vi "fastReadFrames.vi"() -> ()   [LabVIEW 2019]
uses:
  <vilib>/myRIO/Instrument Drivers/Onboard IO/AI/typedefs/AI Reference.ctl
  <vilib>/myRIO/Common/Instrument Driver Framework/Utilities/typedefs/myRIO Generic Hardware Reference.ctl
  <vilib>/myRIO/Common/Instrument Driver Framework/Utilities/typedefs/Hardware Version Enum.ctl
  <vilib>/myRIO/Common/Instrument Driver Framework/Utilities/typedefs/myRIO v1.0 Reference.ctl
  <vilib>/myRIO/Common/Instrument Driver Framework/Utilities/typedefs/Generic FPGA Reference.ctl
  <vilib>/myRIO/Common/Instrument Driver Framework/myRIO v1.0/AI/typedefs/AI Channels List.ctl
  <vilib>/myRIO/Common/Instrument Driver Framework/myRIO v1.0/AI/typedefs/AI Channels Enum.ctl
  <vilib>/myRIO/Common/Instrument Driver Framework/Utilities/typedefs/Analog Scaling Constants List.ctl
  <vilib>/myRIO/Common/Instrument Driver Framework/Utilities/typedefs/Analog Scaling Constants.ctl
  <vilib>/userdefined/High Color/nirio_resource_hc.ctl
  <vilib>/Platform/TimedLoop/XDataNode/timing_clust.ctl
  <vilib>/Platform/TimedLoop/XDataNode/nitl_modes.ctl
  <vilib>/Platform/TimedLoop/XDataNode/wakeup.ctl
  <vilib>/myRIO/Common/Instrument Driver Framework/myRIO v1.0/AI/vis/myRIO v1.1 Open Throughput AI.vi
  <vilib>/Analysis/baseanly.llb/Mean (DBL).vi
  <vilib>/myRIO/Common/Instrument Driver Framework/Utilities/vis/Validate Channels.vi
  <vilib>/myRIO/Common/Instrument Driver Framework/myRIO v1.0/AI/vis/myRIO v1.0 Reserve AI.vi
  <vilib>/myRIO/Common/Instrument Driver Framework/myRIO v1.0/AI/vis/myRIO v1.0 Close AI.vi
  <vilib>/myRIO/Common/Instrument Driver Framework/myRIO v1.0/AI/vis/myRIO v1.0 Build MUX Configuration AI.vi
  <vilib>/myRIO/Common/Instrument Driver Framework/myRIO v1.0/Resource Manager/vis/myRIO v1.0 Reserve Channel List.vi
  <vilib>/myRIO/Common/Instrument Driver Framework/myRIO v1.0/AI/vis/myRIO v1.0 Unreserve AI.vi
  <vilib>/myRIO/Common/Instrument Driver Framework/myRIO v1.0/Resource Manager/vis/myRIO v1.0 Reserve Channel.vi
  <vilib>/myRIO/Common/Instrument Driver Framework/myRIO v1.0/Resource Manager/vis/myRIO v1.0 Unreserve Channel.vi
  <vilib>/myRIO/Common/Instrument Driver Framework/myRIO v1.0/Resource Manager/vis/myRIO v1.0 Unreserve Channel List.vi
  <vilib>/myRIO/Common/Instrument Driver Framework/myRIO v1.0/Resource Manager/vis/myRIO v1.0 Build Mutex Name.vi
  <vilib>/Utility/VariantDataType/GetNumericInfo.vi
  <vilib>/Utility/error.llb/Error Cluster From Error Code.vi
  <vilib>/myRIO/Common/Instrument Driver Framework/myRIO v1.0/myRIO v1.1 Open Throughput.vi
  <vilib>/myRIO/Common/Instrument Driver Framework/myRIO v1.0/AI/vis/myRIO v1.0 Get Scaling Constants AI.vi
  <vilib>/myRIO/Common/Instrument Driver Framework/Utilities/vis/IO Manager.vi
  <vilib>/myRIO/Common/Instrument Driver Framework/Utilities/vis/Configuration Manager.vi
  <vilib>/myRIO/Common/Instrument Driver Framework/myRIO v1.0/myRIO v1.0 Close.vi
  <vilib>/myRIO/Common/Instrument Driver Framework/myRIO v1.0/AI/vis/myRIO v1.0 Read AI.vi
  <vilib>/myRIO/Instrument Drivers/Onboard IO/AI/vis/myRIO AI Open.xnode
  <vilib>/platform/TimedLoop/XDataNode/XDataNode.xnode
  <vilib>/Platform/TimedLoop/XDataNode/XDNodeRunTimeDep.lvlib
  <vilib>/myRIO/Instrument Drivers/Onboard IO/AI/AI.lvlib
  <vilib>/Analysis/NI_AALBase.lvlib
panel:
  out "dt":dbl[](graph)
  out "puste?":bool[](array[boolean])
  out "size(s)":i32[](array[numeric])
  in  "Frame length ms":i64=50
  out "dt ramki":u32
  out "Waveform Chart":dbl[][](graph)
  in  "stop":bool
  in  "Channel Names":tag[](array[tag])=["B/AI0", "B/AI1", "B/AI2"]
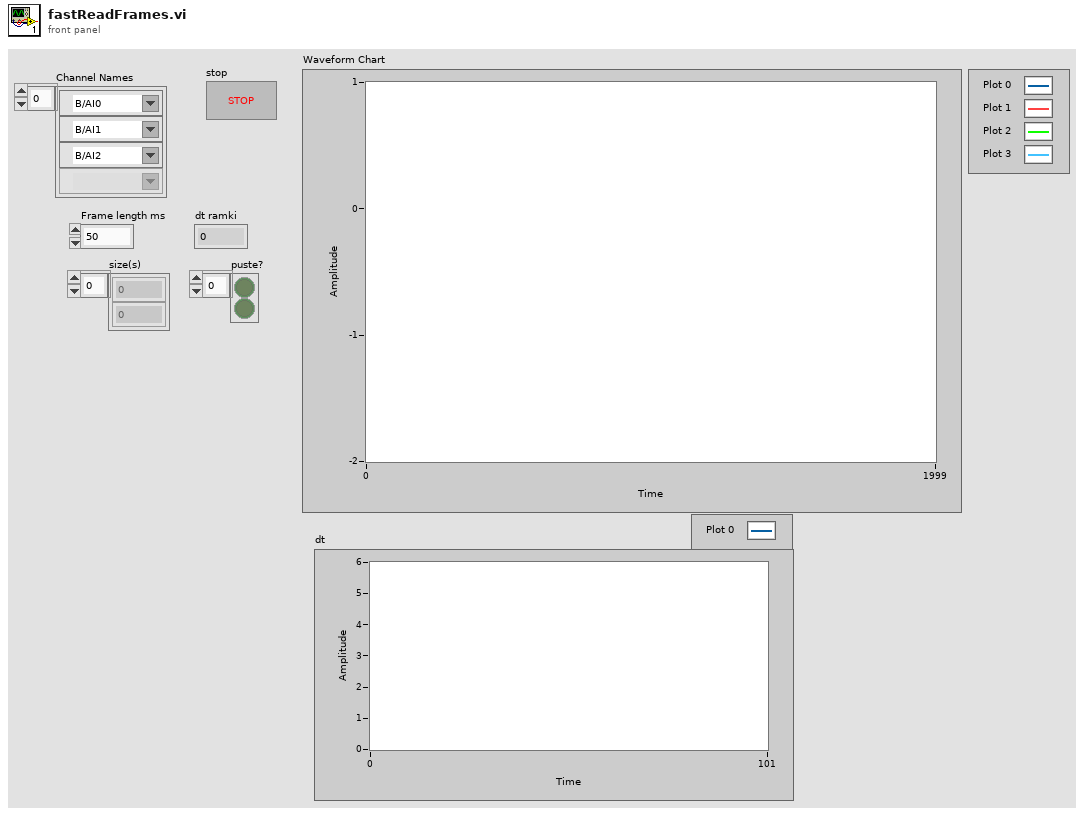
[diagram p1: front panel]
types:
  T1 = typedef "nirio_resource_hc.ctl" = tag
  T2 = typedef "Hardware Version Enum.ctl" = enum16{"Unknown", "myRIO-1900", "myRIO-1950", "roboRIO", "NI ELVIS RIO CM", "ELVIS III"}
  T3 = typedef "AI.lvlib/AI Reference.ctl" = cluster{"myRIO Reference":T4, "AI Channels List":T7, "AI Scaling Constants List":T9}
  T4 = typedef "myRIO Generic Hardware Reference.ctl" = cluster{"myRIO Model":T2, "myRIO Hardware Reference":T5}
  T5 = typedef "myRIO v1.0 Reference.ctl" = cluster{"Generic FPGA Reference":T6, "Allow multiple opens":bool}
  T6 = typedef "Generic FPGA Reference.ctl" = refnum<k20>
  T7 = typedef "AI Channels List.ctl" = T8[]
  T8 = typedef "AI Channels Enum.ctl" = enum16{"Not Connected", "AudioIn/Left", "AudioIn/Right", "C/AI0", "C/AI1", "A/AI0", "A/AI1", "A/AI2", "A/AI3", "A/AI4", "A/AI5", "A/AI6", "A/AI7", "B/AI0", "B/AI1", "B/AI2", "B/AI3", "B/AI4", "B/AI5", "B/AI6", "B/AI7", "AI/AI0", "AI/AI1", "AI/AI2", "AI/AI3", "A/AI0 (DIFF)", "A/AI1 (DIFF)", "A/AI2 (DIFF)", "A/AI3 (DIFF)", "B/AI0 (DIFF)", "B/AI1 (DIFF)", "B/AI2 (DIFF)", "B/AI3 (DIFF)"}
  T9 = typedef "Analog Scaling Constants List.ctl" = T10[]
  T10 = typedef "Analog Scaling Constants.ctl" = cluster{"LSB Weight (Volts)":dbl, "Offset (Volts)":dbl, "Signed?":bool}
  T11 = typedef "XDNodeRunTimeDep.lvlib/timing_clust.ctl" = cluster{"Expected End [f-1]":u64, "Actual End [f-1]":u64, "Finished Late? [f-1]":bool, "Expected End [i-1]":u64, "Actual End [i-1]":u64, "Finished Late? [i-1]":bool, "Expected Start [i]":u64, "Actual Start [i]":u64, "Expected Start [f]":u64, "Actual Start [f]":u64, "Source Name":string, "Structure Name":string, "Period":i64, "Deadline":i64, "Offset":i64, "Start":i64, "Priority":i32, "Timeout":i32, "Mode":T12, "Wakeup Reason":T13, "Error":errorcluster, "Source Type":string, "Secondary Source Type":string, "Global End Time":u64, "Global Start Time":u64, "Frame Duration":u64, "Iteration Duration":u64, "Assigned CPU":i32, "I/O Scan Engine Mode":u32}
  T12 = typedef "XDNodeRunTimeDep.lvlib/nitl_modes.ctl" = enum32{"No Change", "Process missed periods, maintain original phase", "Discard missed periods, maintain original phase", "Process missed periods, ignore original phase", "Discard missed periods, ignore original phase"}
  T13 = typedef "XDNodeRunTimeDep.lvlib/wakeup.ctl" = enum32{"Normal", "Aborted", "Asynchronous wakeup", "Timing source error", "Timed loop error", "Timeout"}
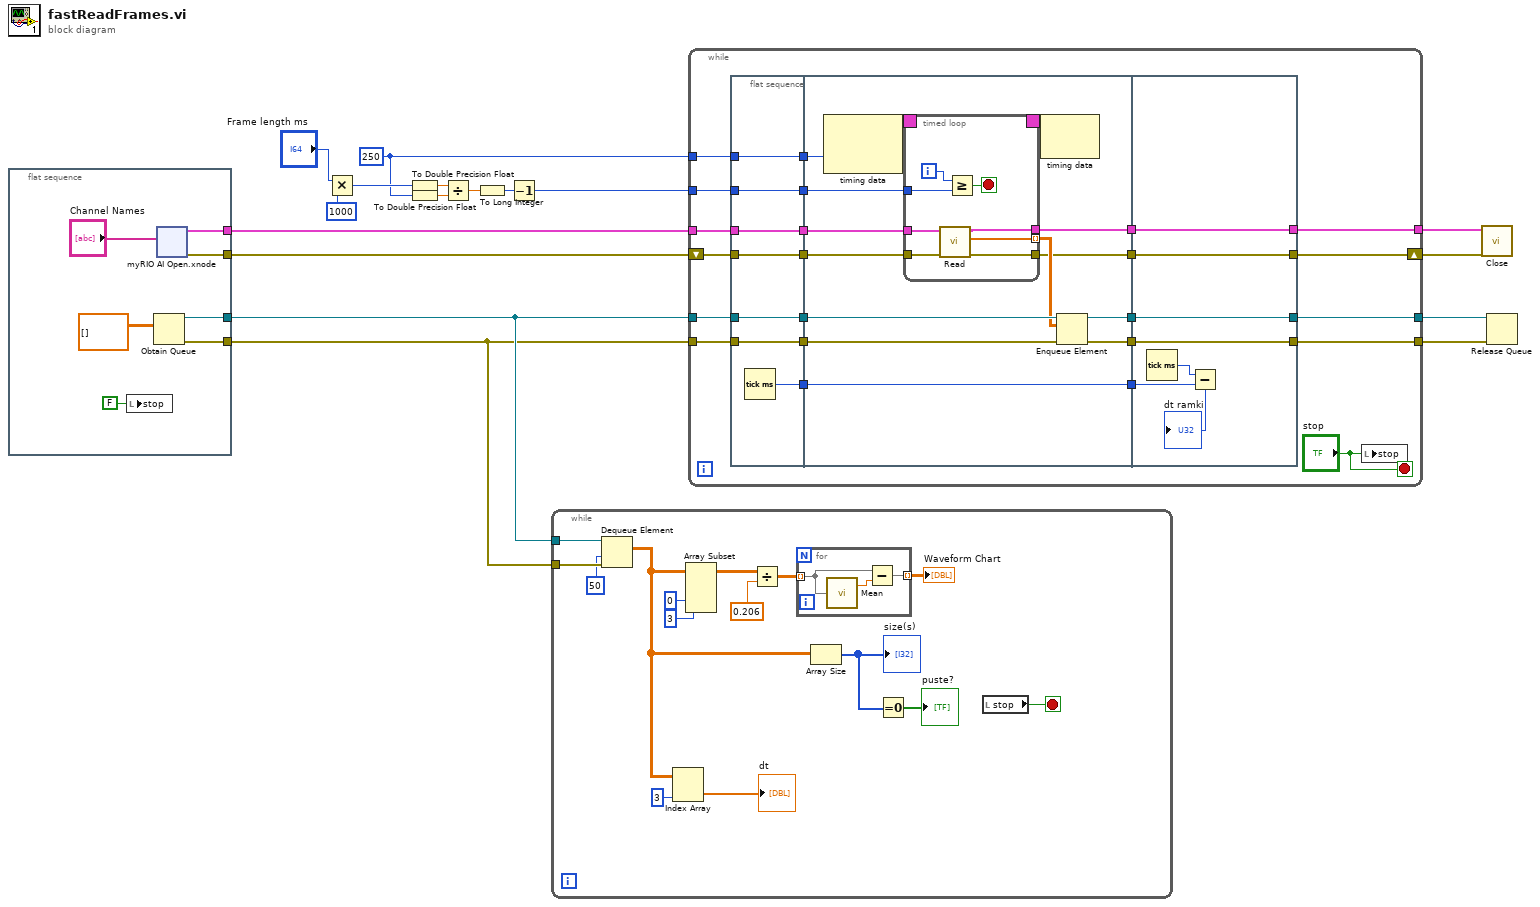
[diagram p0: block diagram]
diagram:
  w3 = i64 250 ("Period")
  n1 = flat-sequence {
    tunnel: [w24] -> w17
    tunnel: [w23] -> w16
    tunnel: [w20] -> w13
    tunnel: [w19] -> w12
    frame #0 {
      n2 = local write "stop"(FALSE ("stop")) -> ()
      n3 = Obtain Queue(element data type=dbl[][] [] ("Values")) -> (queue out=w20:refnum<queue>, error out=w19:errorcluster)  [unwired: 4 in, 1 out]
      n4 = xnode "myRIO AI Open.xnode"("Channel Names"="Channel Names") -> ("error out"=w23:errorcluster, "AI Ref Out"=w24:T3)  [unwired: 2 in]
    }
  }
  n5 = Multiply(x="Frame length ms", y=i64 1000) -> (x*y=w5:i64)
  n6 = To Double Precision Float(number=w5) -> (double precision float=w6:dbl)
  n7 = To Double Precision Float(number=w3) -> (double precision float=w7:dbl)
  n8 = Divide(x=w6, y=w7) -> (x/y=w8:dbl)
  n9 = To Long Integer(number=w8) -> (32bit integer=w9:i32)
  n10 = Decrement(x=w9) -> (x-1=w2:i32)
  n11 = while {
    tunnel: w13 -> [w57]
    tunnel: w12 -> [w56]
    stop <- w54 stop-if-true
    n12 = Dequeue Element(queue=w57, timeout in ms (-1)=50, error in (no error)=w56) -> (element=w45:dbl[][])  [unwired: 3 out]
    n13 = Index Array(array=w45, index (col)=3 ("disabled index (col)")) -> (element=→"dt":dbl[])  [unwired: 1 in]
    n14 = Array Subset(array=w45, index (col)=0 ("index"), length (col)=3 ("length")) -> (w48:dbl[][])  [unwired: 2 in]
    n15 = Divide(x=w48, y=0.206) -> (x/y=w50:dbl[][])
    n16 = for {
      tunnel: w50 -> [w60] mode=indexing
      tunnel: [w59] -> w49 mode=indexing
      n17 = call-poly <vilib>:"Mean.vi"("X"=w60) -> ("mean"=w58:dbl)  [unwired: 1 out]
      n18 = Subtract(x=w60, y=w58) -> (x-y=w59:dbl[])
    }
    "Waveform Chart" <- w49
    n19 = Array Size(array=w45) -> (size(s)=w53:i32[])
    "size(s)" <- w53
    n20 = Equal To 0?(x=w53) -> (x = 0?=→"puste?":bool[])
    n21 = local read "stop"() -> (w54:bool)
  }
  n22 = while {
    tunnel: w17 -> [w83]
    tunnel: w13 -> [w81]
    tunnel: w12 -> [w80]
    tunnel: [w79] -> w15
    tunnel: [w78] -> w14
    tunnel: [w76] -> w11
    shift-right: [w75] -> w10
    shift-left: w16 -> [w82]
    tunnel: w3 -> [w63]
    tunnel: w2 -> [w61]
    stop <- "stop" stop-if-true
    n23 = flat-sequence {
      tunnel: w80 -> [w87]
      tunnel: w81 -> [w88]
      tunnel: w82 -> [w89]
      tunnel: w83 -> [w90]
      tunnel: [w90] -> w74
      tunnel: [w89] -> w73
      tunnel: [w88] -> w72
      tunnel: [w87] -> w71
      tunnel: [w86] -> w70
      tunnel: [w85] -> w64
      tunnel: w63 -> [w85]
      tunnel: [w84] -> w62
      tunnel: w61 -> [w84]
      tunnel: w74 -> [w102]
      tunnel: w73 -> [w101]
      tunnel: w72 -> [w100]
      tunnel: w71 -> [w99]
      tunnel: w70 -> [w93]
      tunnel: [w97] -> w69
      tunnel: [w96] -> w68
      tunnel: [w95] -> w67
      tunnel: [w94] -> w66
      tunnel: [w93] -> w65
      tunnel: w64 -> [w92]
      tunnel: w62 -> [w91]
      tunnel: [w122] -> w75
      tunnel: [w123] -> w76
      tunnel: [w124] -> w78
      tunnel: [w125] -> w79
      tunnel: w69 -> [w125]
      tunnel: w68 -> [w124]
      tunnel: w67 -> [w123]
      tunnel: w66 -> [w122]
      tunnel: w65 -> [w121]
      frame #0 {
        n24 = Tick Count (ms)() -> (millisecond timer value=w86:u32)
      }
      frame #1 {
        n25 = node-c288(w92) -> (w104:T11)  [unwired: 1 in]
        n26 = timed-loop {
          timing: w104 -> [_]
          timing-out: [_] -> w103
          tunnel: w102 -> [w110]
          tunnel: w101 -> [w109]
          tunnel: [w108] -> w95
          tunnel: [w107] -> w94
          tunnel: [w106] -> w98 mode=indexing
          tunnel: w91 -> [w105]
          i -> [w111]
          stop <- w112 stop-if-true
          n27 = call <vilib>:"Read.vi"("error in (no error)"=w109, "AI Ref In"=w110) -> ("error out"=w107:errorcluster, "Values"=w106:dbl[], "AI Ref Out"=w108:T3)  [unwired: 7 in]
          n28 = Greater Or Equal?(x=w111, y=w105) -> (x >= y?=w112:bool)
        }
        n29 = node-c288(w103) -> ()  [unwired: 1 out]
        n30 = Enqueue Element(queue=w100, element=w98, error in (no error)=w99) -> (queue out=w97:refnum<queue>, error out=w96:errorcluster)  [unwired: 1 in, 1 out]
      }
      frame #2 {
        n31 = Tick Count (ms)() -> (millisecond timer value=w120:u32)
        n32 = Subtract(x=w120, y=w121) -> (x-y=→"dt ramki":u32)
      }
    }
    n33 = local write "stop"("stop") -> ()
  }
  n34 = call <vilib>:"Close.vi"("error in (no error)"=w10, "AI Ref In"=w11) -> ()  [unwired: 9 in, 1 out]
  n35 = Release Queue(queue=w15, error in (no error)=w14) -> ()  [unwired: 1 in, 3 out]
